vi "ErrorMSG_UI Control Reference.vi"(7 "Function":enum16{"read", "write"}(ring), 8 "error in":errorcluster, 11 "RefIn":cluster{"Main_Tab":refnum<vi>}) -> (0 "error out":errorcluster, 3 "RefOut":cluster{"Main_Tab":refnum<vi>})   [LabVIEW 2019]
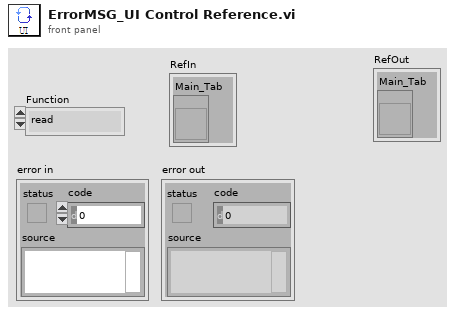
[diagram p1: front panel]
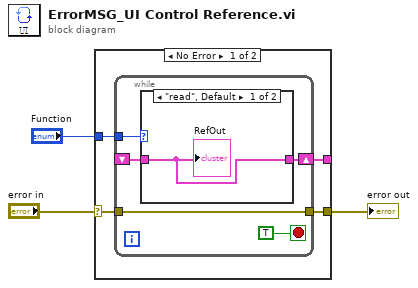
[diagram p0: block diagram]
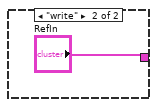
[diagram p2: hidden frame]
diagram:
  n1 = case shown="No Error" "error in" {
    selector: "error in" -> [w5 w15]
    tunnel: "Function" -> [w7 _]
    tunnel: [w6 w15] -> w1
    tunnel: [w4 _] -> _
    frame No Error {
      n2 = while {
        shift-right: [w10] -> w4
        shift-left: _ -> [w8]
        tunnel: w7 -> [w11]
        tunnel: [w9] -> w6
        tunnel: w5 -> [w9]
        stop <- TRUE stop-if-true
        n3 = case shown="\"read\", Default" w11 {
          tunnel: [w13 "RefIn"] -> w10
          tunnel: w8 -> [w13 _]
          frame "read", Default {
            "RefOut" <- w13
          }
          frame "write" {
          }
        }
      }
    }
    frame Error {
    }
  }
  "error out" <- w1
